vi "Write BMP File.vi"(8 "error in (no error)":errorcluster, 10 "image data":T1, 11 "path to BMP file":path) -> (0 "error out":errorcluster, 3 "path":path)   [LabVIEW 2020]
doc: "Writes a Windows bitmap file."
uses:
  imagedata.ctl
panel:
  in  "Select the BMP file to write":string="Select the BMP file to write"
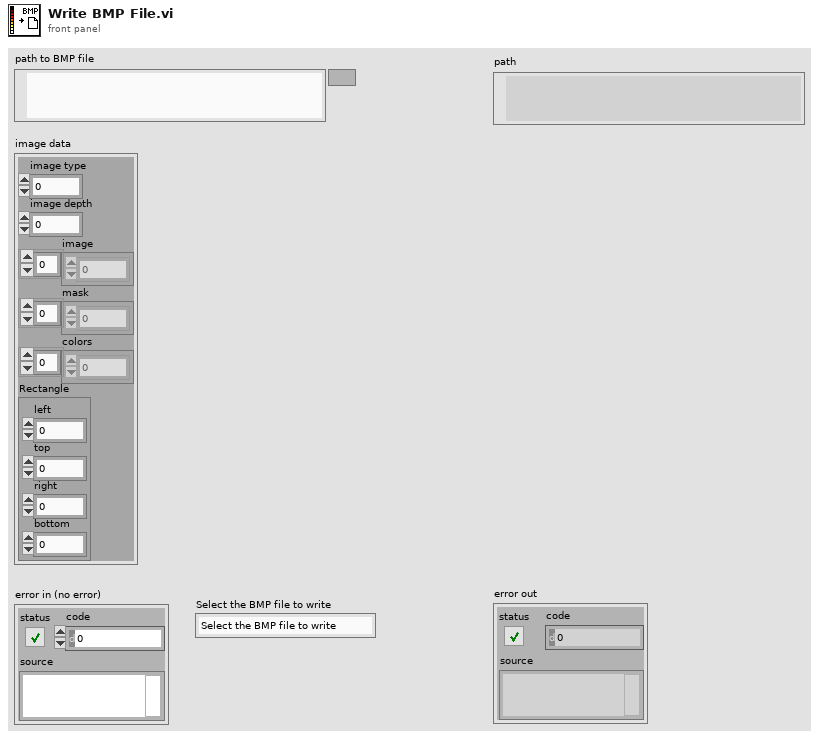
[diagram p1: front panel]
types:
  T1 = typedef "imagedata.ctl" = cluster{"image type":i32, "image depth":i32, "image":u8[], "mask":u8[], "colors":u32[], "Rectangle":cluster{"left":i16, "top":i16, "right":i16, "bottom":i16}}
  T2 = cluster{"sizeof header":u32, "width":u32, "height":u32, "planes":u16, "bpp":u16, "compression":u32, "byte size":u32, "horiz res":u32, "vert res":u32, "colors used":u32, "colors important":u32}
  T3 = enum16{"open", "replace", "create", "open or create", "replace or create", "replace or create with confirmation"}
  T4 = cluster{"left":i16, "top":i16, "right":i16, "bottom":i16}
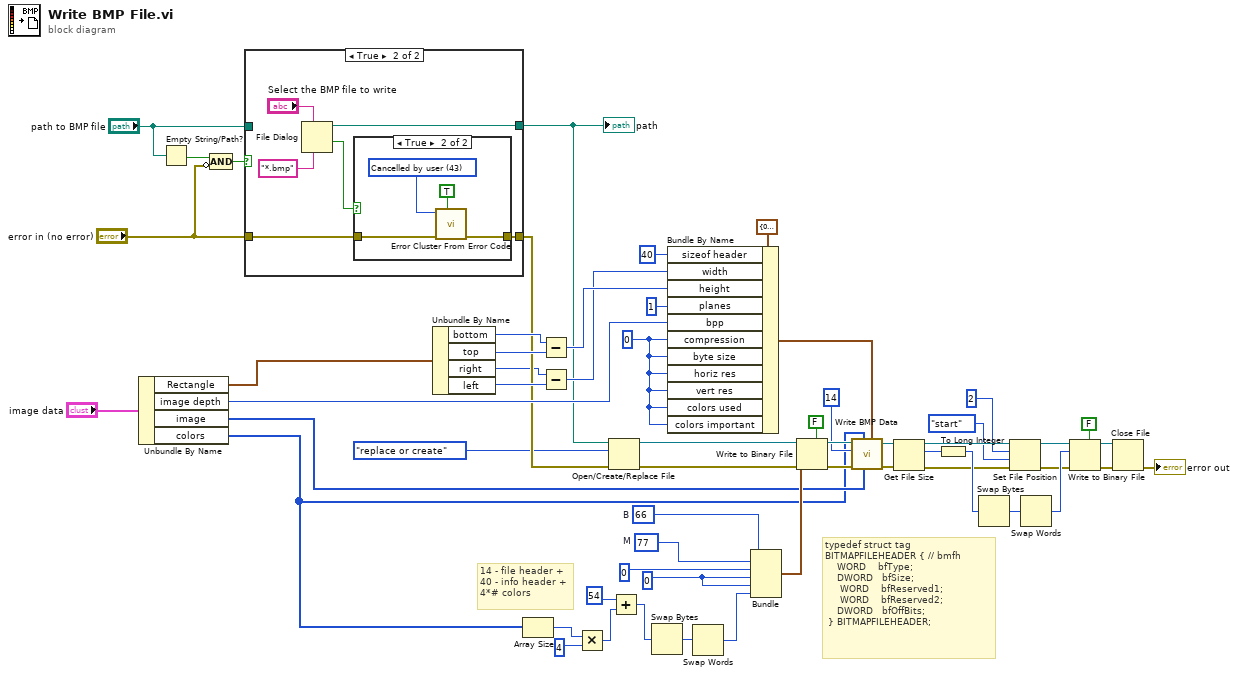
[diagram p0: block diagram]
diagram:
  w44 = u8 77  # M
  w42 = u8 66  # B
  w29 = u16 0
  w2 = u32 0 ("compression")
  # "typedef struct tag\nBITMAPFILEHEADER { // bmfh    \n    WORD    bfType; \n    DWORD   bfSize;\n     WORD    bfReserved1;\n     WORD    bfReserved2; \n    DWORD   bfOffBits;\n } BITMAPFILEHEADER;"
  # "14 - file header +\n40 - info header +\n4*# colors"
  n1 = Unbundle By Name("image data") -> ("Rectangle"=w3:T4, "image depth"=w22:i32, "image"=w21:u8[], "colors"=w20:u32[])
  n2 = Empty String/Path?(string/path="path to BMP file") -> (empty?=w18:bool)
  n3 = Compound Arithmetic op=AND(w18, invert "error in (no error)") -> (w19:bool)
  n4 = case shown="True" w19 {
    tunnel: [w59 w64] -> w14
    tunnel: "path to BMP file" -> [w59 _]
    tunnel: "error in (no error)" -> [w58 w62]
    tunnel: [w58 w61] -> w16
    frame False {
    }
    frame True {
      n5 = File Dialog(6:"*.bmp", 7:"Select the BMP file to write") -> (1:w63:bool, 3:w64:path)  [unwired: 5 in, 2 out]
      n6 = case shown="True" w63 {
        tunnel: w62 -> [w66 w70]
        tunnel: [w66 w69] -> w61
        frame False {
        }
        frame True {
          w67 = u16 43 items=["No error", "Argument error", "Memory is full", "Out of zone", "End of file", "File already open", "Generic file I/O error", "File not found", "File permission error", "Disk is full", "Duplicate path", "Too many files open", "System feature not enabled", "Resource file not found", "Cannot add resource", "Resource not found", "Image not found", "Image memory error", "Pen does not exist", "Config type invalid", "Config token not found", "Config parse error", "Config memory error", "Bad external code format", "Bad external code offset", "External code not present", "Null window", "Destroy window error", "Null menu", "Print aborted", "Bad print record", "Print driver error", "Windows error during printing", "Memory error during printing", "Print dialog error", "Generic print error", "Invalid device refnum", "Device not found", "Device parameter error", "Device unit error", "Cannot open device", "Device call aborted", "Generic error", "Cancelled by user", "Object ID too low", "Object ID too high", "Object not in heap", "Unknown heap", "Unknown object (invalid DefProc)", "Unknown object (DefProc not in table)", "Message out of range", "Invalid (null) method", "Unknown message", "Manager call not supported", "Bad address", "Network operation in progress", "Network operation timed out", "Connection is busy", "Network attribute not supported", "Network error", "Address in use", "System out of memory", "Connection aborted", "Connection refused", "Not connected", "Already connected", "Connection closed", "Initialization error (interapplication manager)", "Bad occurrence", "Wait on unbound occurrence handler", "Occurrence queue overflow", "Datalog type conflict", "Unused", "Unrecognized type (interapplication manager)", "Memory corrupt", "Failed to make temporary DLL", "Old CIN version", "Drag socket not found", "Failed to load drop-object", "Failed to register OLE object", "Failed to release OLE object", "Format specifier type mismatch", "Unknown format specifier", "Too few format specifiers", "Too many format specifiers", "Scan failed", "Newer CIN version", "OLE Convert", "Runtime menu error", "Password tampered", "Unknown error code"]
          n7 = call "Error Cluster From Error Code.vi"("show call chain? (False)"=TRUE, "error in (no error)"=w70, "error code (0)"=w67) -> ("error out"=w69:errorcluster)  [unwired: 6 in]
        }
      }
    }
  }
  "path" <- w14
  n8 = Unbundle By Name(w3) -> ("bottom"=w55:i16, "top"=w54:i16, "right"=w1:i16, "left"=w53:i16)
  n9 = Array Size(array=w20) -> (size(s)=w28:i32)
  n10 = Subtract(x=w55, y=w54) -> (x-y=w25:i16)
  n11 = Subtract(x=w1, y=w53) -> (x-y=w24:i16)
  n12 = Multiply(x=w28, y=4) -> (x*y=w26:i32)
  n13 = Open/Create/Replace File(file path (use dialog)=w14, error in=w16, operation (0:open)=T3."replace or create") -> (refnum out=w46:refnum<file>, error out=w47:errorcluster)  [unwired: 3 in, 1 out]
  n14 = Add(x=54, y=w26) -> (x+y=w40:i32)
  n15 = Swap Bytes(anything=w40) -> (byte swapped=w41:i32)
  n16 = Bundle By Name(cluster=T2 {"sizeof header"=0, "width"=0, "height"=0, "planes"=0, "bpp"=0, "compression"=0, "byte size"=0, "horiz res"=0, "vert res"=0, "colors used"=0, "colors important"=0} ("bmp header"), "sizeof header"=u32 40, "width"=w24, "height"=w25, "planes"=u16 1, "bpp"=w22, "compression"=w2, "byte size"=w2, "horiz res"=w2, "vert res"=w2, "colors used"=w2, "colors important"=w2) -> (w56:T2)
  n17 = Swap Words(1:w41) -> (0:w39:i32)
  n18 = Bundle("B"=w42, "M"=w44, 0, w29, w29, w39) -> (w38:cluster{"B":u8, "M":u8, i32, u16, u16, i32})  [unwired: 1 in]
  n19 = Write to Binary File(file (use dialog)=w46, data=w38, error in=w47, 5:FALSE ("prepend array or string size? (T)")) -> (refnum out=w48:refnum<file>, error out=w49:errorcluster)  [unwired: 2 in, 1 out]
  n20 = call "Write BMP Data.vi"("bmp header"=w56, "data"=w21, "color table"=w20, "error in (no error)"=w49, "offset"=14, "file path"=w48) -> ("error out"=w37:errorcluster, "file path copy"=w36:refnum<file>)  [unwired: 4 in]
  n21 = Get File Size(file=w36, error in=w37) -> (refnum out=w31:refnum<file>, size (in bytes)=w13:i64, 0:w30:errorcluster)
  n22 = To Long Integer(number=w13) -> (32bit integer=w32:i32)
  n23 = Swap Bytes(anything=w32) -> (byte swapped=w11:i32)
  n24 = Set File Position(offset (in bytes) (0)=2 ("pos offset (0)"), refnum=w31, from (0:start)=enum16{"start", "end", "current"}."start" ("pos mode (0:2)"), error in=w30) -> (refnum out=w7:refnum<file>, error out=w6:errorcluster)
  n25 = Swap Words(1:w11) -> (0:w10:i32)
  n26 = Write to Binary File(file (use dialog)=w7, data=w10, error in=w6, 5:FALSE ("prepend array or string size? (T)")) -> (refnum out=w35:refnum<file>, error out=w34:errorcluster)  [unwired: 2 in, 1 out]
  n27 = Close File(refnum=w35, error in=w34) -> (error out=→"error out":errorcluster)  [unwired: 1 out]
